vi "Is Color Transparent.vi"(2 "original color":u32(colorbox), 4 "desired color":u32(colorbox)) -> (5 "updated color":u32(colorbox))   [LabVIEW 2026, in "TSC Material Theme.lvlib" / "Material-Scheme.lvclass"]
doc: "check if original was transparent, if so, don't change it, if it isn't though, pass out the new color\n\n<b>Code Developed By:</b> +\nDaniel Coons +\nTechnology Service Corporation +\nwww.tsc.com/atcs"
uses:
  Material-Scheme.lvclass
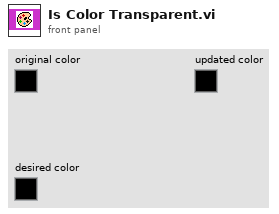
[diagram p1: front panel]
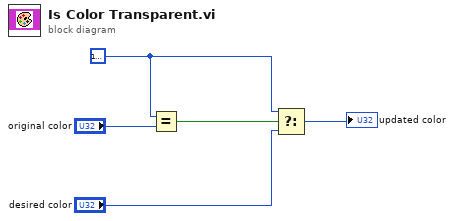
[diagram p0: block diagram]
diagram:
  w3 = u32 16777216
  n1 = Equal?(x=w3, y="original color") -> (x = y?=w4:bool)
  n2 = Select(t=w3, s=w4, f="desired color") -> (s? t:f=→"updated color":u32)
